vi "Modified Bessel Function Iv.vi"(2 "v":dbl format="%.2f", 3 "x":dbl format="%.2f") -> (1 "Iv(x)":dbl format="%.2f")   [LabVIEW 2020, in "NI_Gmath.lvlib"]
doc: "Computes the modified Bessel function of the first kind."
uses:
  <vilib>/gmath/NI_Gmath.lvlib
  <resource>/lvanlys.dll
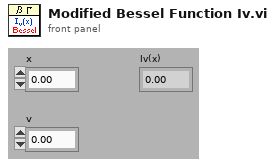
[diagram p1: front panel]
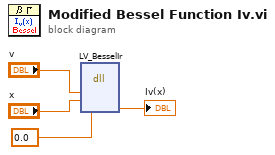
[diagram p0: block diagram]
diagram:
  n1 = dll-call lib="e:/builds/penguin/labview/branches/2020/dev/dist/resource/lvanlys.*" fn="LV_BesselIr"("v"="v", "x"="x", "Iv(x)"=0.0 ("Jr")) -> ("Iv(x)"=→"Iv(x)":dbl)  [unwired: 6 in, 2 out]
